vi "poly_time_conversion_s2ms_array.vi"(2 "s":dbl[](array[numeric]) format="%#_13g") -> (7 "ms":i32[](array[numeric]))   [LabVIEW 2015]
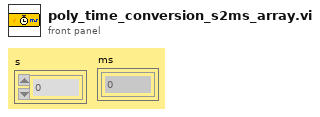
[diagram p1: front panel]
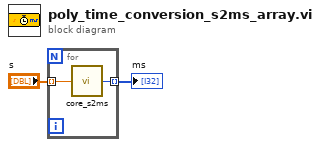
[diagram p0: block diagram]
diagram:
  n1 = for {
    tunnel: "s" -> [w4] mode=indexing
    tunnel: [w3] -> w1 mode=indexing
    n2 = call "core_s2ms.vi"("s {DBL}"=w4) -> ("ms {I32}"=w3:i32)  [unwired: 8 in]
  }
  "ms" <- w1
